vi "UpdateComm.vi"(8 "error in (no error)":errorcluster, 11 "Acquisition in":refnum<class "Acquisition.lvclass">) -> (0 "error out":errorcluster, 3 "Acquisition out":refnum<class "Acquisition.lvclass">)   [LabVIEW 2018, in "Acquisition.lvclass"]
uses:
  Acquisition.lvclass
  C:/Users/devstaff/sparc4/s4gui/Versao ZeroMQ REQ-REP/SPARC4_GUI -20240801_20240708/Server/Server.lvclass
  Acquisition.lvclass/Acquisition.ctl
  Device/Device.lvclass/Device.ctl
  Server/Server.lvclass/Server.ctl
  Interface/Interface.lvclass/Interface.ctl
  Channel/Channel.lvclass
  C:/Users/devstaff/sparc4/s4gui/Versao ZeroMQ REQ-REP/SPARC4_GUI -20240801_20240708/Device/Device.lvclass
  Server/Server.lvclass
  Device/Device.lvclass
  StateMachine/State Machine.lvclass
  Interface/Interface.lvclass
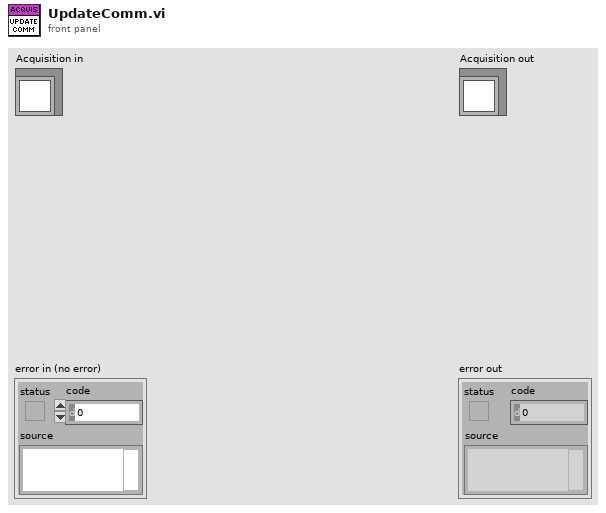
[diagram p1: front panel]
types:
  T1 = cluster{"ACQUISITION_MODE":bool, "TRIGGER_MODE":bool, "READ_MODE":bool, "PREAMP":bool, "READOUT_RATE":bool, "VERTICAL_SHIFT_SPEED":bool, "EM_MODE":bool, "EM_GAIN":bool, "SHUTTER_MODE":bool, "SHUTTER_TTL":bool, "SHUTTER_OPENING_TIME":bool, "SHUTTER_CLOSING_TIME":bool, "VBIN":bool, "HBIN":bool, "INITIAL_LINE":bool, "INITIAL_COLUMN":bool, "FINAL_LINE":bool, "FINAL_COLUMN":bool, "FRAME_TRANSFER":bool, "VERTICAL_CLOCK_VOLTAGE":bool, "AD_CHANNEL":bool}
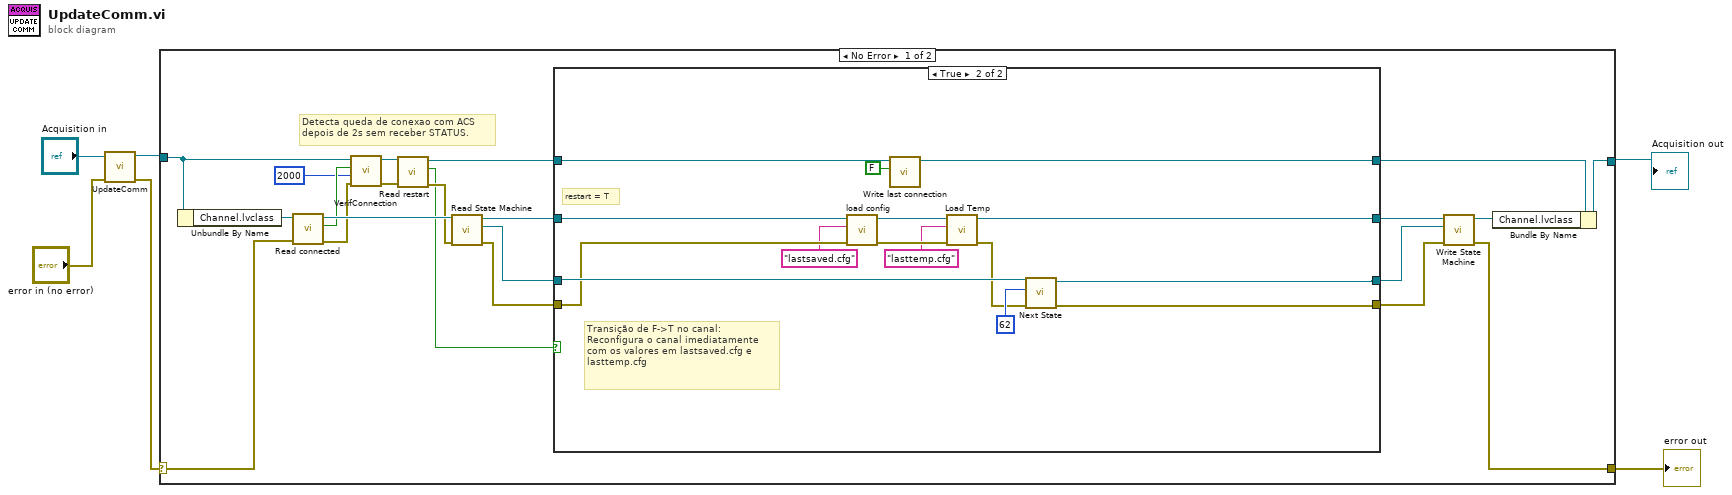
[diagram p0: block diagram]
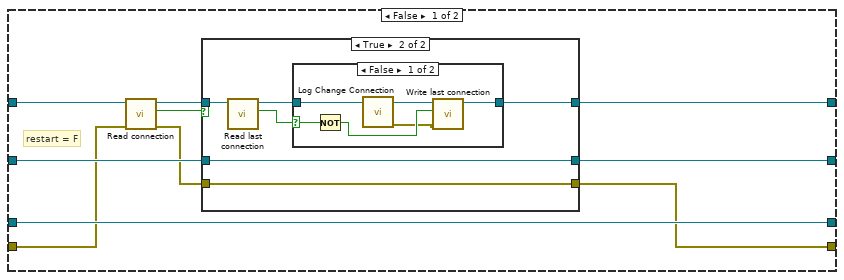
[diagram p2: hidden frame]
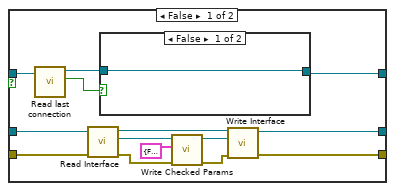
[diagram p3: hidden frame]
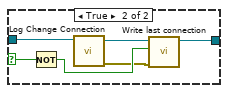
[diagram p4: hidden frame]
diagram:
  n1 = call-parent "UpdateComm.vi"("error in (no error)"="error in (no error)", "Server in"="Acquisition in") -> ("error out"=w3:errorcluster, "Server out"=w4:refnum<class "Acquisition.lvclass">)  [unwired: 8 in]
  n2 = case shown="No Error" w3 {
    selector: w3 -> [w27 w89]
    tunnel: [w19 w89] -> w1
    tunnel: [w20 w88] -> w2
    tunnel: w4 -> [w22 w88]
    frame No Error {
      # "Detecta queda de conexao com ACS\ndepois de 2s sem receber STATUS."
      n3 = Unbundle By Name(w22) -> ("Channel.lvclass"=w28:refnum<class "Channel.lvclass">)
      n4 = call "Read connected.vi"("error in (no error)"=w27, "Device in"=w28) -> ("error out"=w21:errorcluster, "connected"=w12:bool, "Device out"=w26:refnum<class "Channel.lvclass">)  [unwired: 7 in]
      n5 = call-dynamic "VerifConnection.vi"("error in (no error)"=w21, "timeout in ms (1000)"=u32 2000, "device connected in"=w12, "Server in"=w22) -> ("error out"=w17:errorcluster, "Server out"=w18:refnum<class "Acquisition.lvclass">)  [unwired: 6 in]
      n6 = call-dynamic "Read restart.vi"("error in (no error)"=w17, "Server in"=w18) -> ("error out"=w16:errorcluster, "restart"=w15:bool, "Server out"=w9:refnum<class "Acquisition.lvclass">)  [unwired: 7 in]
      n7 = call-dynamic "Read State Machine.vi"("error in (no error)"=w16, "Device in"=w26) -> ("error out"=w10:errorcluster, "State Machine.lvclass"=w11:refnum<class "State Machine.lvclass">, "Device out"=w14:refnum<class "Channel.lvclass">)  [unwired: 7 in]
      n8 = case shown="True" w15 {
        tunnel: w11 -> [w38 w87]
        tunnel: [w38 w82] -> w25
        tunnel: w10 -> [w31 w84]
        tunnel: [w29 w86] -> w24
        tunnel: w14 -> [w33 w85]
        tunnel: [w32 w83] -> w13
        tunnel: [w34 w73] -> w8
        tunnel: w9 -> [w37 w75]
        frame False {
          # "restart = F"
          n9 = call "Read connection.vi"("error in (no error)"=w31, "Server in"=w37) -> ("error out"=w30:errorcluster, "connection"=w36:bool, "Server out"=w35:refnum<class "Acquisition.lvclass">)  [unwired: 7 in]
          n10 = case shown="True" w36 {
            tunnel: [w40 w60] -> w34
            tunnel: w35 -> [w42 w61]
            tunnel: w33 -> [w49 w65]
            tunnel: [w47 w65] -> w32
            tunnel: w30 -> [w51 w64]
            tunnel: [w45 w64] -> w29
            frame False {
              n11 = call-dynamic "Read last connection.vi"("Server in"=w42) -> ("last connection"=w39:bool, "Server out"=w41:refnum<class "Acquisition.lvclass">)  [unwired: 8 in, 1 out]
              n12 = call-dynamic "Read Interface.vi"("error in (no error)"=w51, "Channel in"=w49) -> ("error out"=w50:errorcluster, "Interface.lvclass"=w44:refnum<class "Interface.lvclass">, "Channel out"=w48:refnum<class "Channel.lvclass">)  [unwired: 7 in]
              n13 = case shown="False" w39 {
                selector: w39 -> [_ w56]
                tunnel: w41 -> [w53 w59]
                tunnel: [w53 w57] -> w40
                frame False {
                }
                frame True {
                  n14 = Not(x=w56) -> (.not. x?=w55:bool)
                  n15 = call-dynamic "Log Change Connection.vi"("Server in"=w59) -> ("error out"=w54:errorcluster, "Server out"=w58:refnum<class "Acquisition.lvclass">)  [unwired: 9 in]
                  n16 = call-dynamic "Write last connection.vi"("error in (no error)"=w54, "last connection"=w55, "Server in"=w58) -> ("Server out"=w57:refnum<class "Acquisition.lvclass">)  [unwired: 7 in, 1 out]
                }
              }
              n17 = call "Write Checked Params.vi"("error in (no error)"=w50, "Checked Params"=T1 {"ACQUISITION_MODE"=FALSE, "TRIGGER_MODE"=FALSE, "READ_MODE"=FALSE, "PREAMP"=FALSE, "READOUT_RATE"=FALSE, "VERTICAL_SHIFT_SPEED"=FALSE, "EM_MODE"=FALSE, "EM_GAIN"=FALSE, "SHUTTER_MODE"=FALSE, "SHUTTER_TTL"=FALSE, "SHUTTER_OPENING_TIME"=FALSE, "SHUTTER_CLOSING_TIME"=FALSE, "VBIN"=FALSE, "HBIN"=FALSE, "INITIAL_LINE"=FALSE, "INITIAL_COLUMN"=FALSE, "FINAL_LINE"=FALSE, "FINAL_COLUMN"=FALSE, "FRAME_TRANSFER"=FALSE, "VERTICAL_CLOCK_VOLTAGE"=FALSE, "AD_CHANNEL"=FALSE}, "Interface in"=w44) -> ("error out"=w46:errorcluster, "Interface out"=w43:refnum<class "Interface.lvclass">)  [unwired: 7 in]
              n18 = call-dynamic "Write Interface.vi"("error in (no error)"=w46, "Interface.lvclass"=w43, "Channel in"=w48) -> ("error out"=w45:errorcluster, "Channel out"=w47:refnum<class "Channel.lvclass">)  [unwired: 7 in]
            }
            frame True {
              n19 = call-dynamic "Read last connection.vi"("Server in"=w61) -> ("last connection"=w62:bool, "Server out"=w63:refnum<class "Acquisition.lvclass">)  [unwired: 8 in, 1 out]
              n20 = case shown="False" w62 {
                selector: w62 -> [w68 _]
                tunnel: w63 -> [w71 w72]
                tunnel: [w69 w72] -> w60
                frame False {
                  n21 = Not(x=w68) -> (.not. x?=w67:bool)
                  n22 = call-dynamic "Log Change Connection.vi"("Server in"=w71) -> ("error out"=w66:errorcluster, "Server out"=w70:refnum<class "Acquisition.lvclass">)  [unwired: 9 in]
                  n23 = call-dynamic "Write last connection.vi"("error in (no error)"=w66, "last connection"=w67, "Server in"=w70) -> ("Server out"=w69:refnum<class "Acquisition.lvclass">)  [unwired: 7 in, 1 out]
                }
                frame True {
                }
              }
            }
          }
        }
        frame True {
          # "Transição de F->T no canal:\nReconfigura o canal imediatamente com os valores em lastsaved.cfg e lasttemp.cfg"
          # "restart = T"
          n24 = call-dynamic "load config.vi"("error in (no error)"=w84, "cfg file name"="lastsaved.cfg", "Channel in"=w85) -> ("error out"=w79:errorcluster, "Channel out"=w76:refnum<class "Channel.lvclass">)  [unwired: 7 in]
          n25 = call-dynamic "Write last connection.vi"("last connection"=FALSE, "Server in"=w75) -> ("Server out"=w73:refnum<class "Acquisition.lvclass">)  [unwired: 8 in, 1 out]
          n26 = call-dynamic "Load Temp.vi"("error in (no error)"=w79, "temp file name"="lasttemp.cfg", "Channel in"=w76) -> ("error out"=w78:errorcluster, "Channel out"=w83:refnum<class "Channel.lvclass">)  [unwired: 7 in]
          n27 = call "Next State.vi"("error in (no error)"=w78, "New_State"=62, "State Machine in"=w87) -> ("error out"=w86:errorcluster, "State Machine out"=w82:refnum<class "State Machine.lvclass">)  [unwired: 7 in]
        }
      }
      n28 = call-dynamic "Write State Machine.vi"("error in (no error)"=w24, "State Machine.lvclass"=w25, "Device in"=w13) -> ("error out"=w19:errorcluster, "Device out"=w23:refnum<class "Channel.lvclass">)  [unwired: 7 in]
      n29 = Bundle By Name(cluster=w8, "Channel.lvclass"=w23) -> (w20:refnum<class "Acquisition.lvclass">)
    }
    frame Error {
    }
  }
  "error out" <- w1
  "Acquisition out" <- w2
